vi "MADAQ-SetDACs.vi"(4 "error in (no error)":errorcluster, 5 "DAC 2 [V]":dbl, 6 "DAC  1 [V]":dbl, 7 "VISA resource name":refnum<visa-resource-name>) -> (0 "error out":errorcluster, 3 "VISA resource name out":refnum<visa-resource-name>)   [LabVIEW 2014]
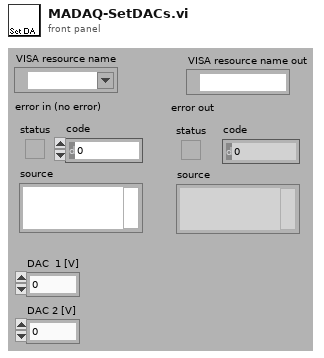
[diagram p1: front panel]
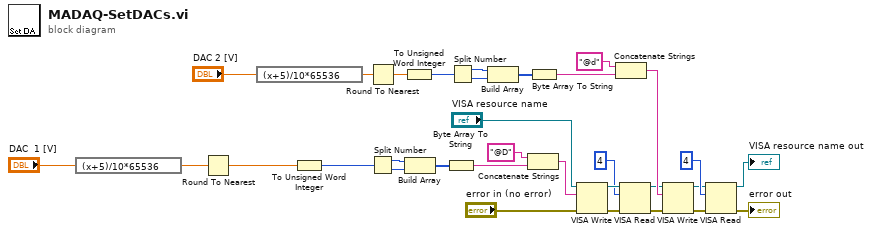
[diagram p0: block diagram]
diagram:
  n1 = expression code="(x+5)/10*65536"("DAC  1 [V]") -> (w8:dbl)
  n2 = Round To Nearest(number=w8) -> (nearest integer value=w7:dbl)
  n3 = expression code="(x+5)/10*65536"("DAC 2 [V]") -> (w6:dbl)
  n4 = To Unsigned Word Integer(number=w7) -> (unsigned 16bit integer=w3:u16)
  n5 = Round To Nearest(number=w6) -> (nearest integer value=w5:dbl)
  n6 = Split Number(x=w3) -> (hi(x)=w32:u8, lo(x)=w31:u8)
  n7 = To Unsigned Word Integer(number=w5) -> (unsigned 16bit integer=w2:u16)
  n8 = Build Array(w32, w31) -> (w28:u8[])
  n9 = Byte Array To String(unsigned byte array=w28) -> (string=w23:string)
  n10 = Split Number(x=w2) -> (hi(x)=w30:u8, lo(x)=w29:u8)
  n11 = Build Array(w30, w29) -> (w27:u8[])
  n12 = Concatenate Strings("@D", w23) -> (w22:string)
  n13 = Byte Array To String(unsigned byte array=w27) -> (string=w11:string)
  n14 = VISA Write(VISA resource name="VISA resource name", write buffer=w22, error in (no error)="error in (no error)") -> (VISA resource name out=w21:refnum<visa-resource-name>, error out=w20:errorcluster)  [unwired: 1 out]
  n15 = Concatenate Strings("@d", w11) -> (w15:string)
  n16 = VISA Read(VISA resource name=w21, byte count=u32 4, error in (no error)=w20) -> (VISA resource name out=w13:refnum<visa-resource-name>, error out=w12:errorcluster)  [unwired: 2 out]
  n17 = VISA Write(VISA resource name=w13, write buffer=w15, error in (no error)=w12) -> (VISA resource name out=w16:refnum<visa-resource-name>, error out=w17:errorcluster)  [unwired: 1 out]
  n18 = VISA Read(VISA resource name=w16, byte count=u32 4, error in (no error)=w17) -> (VISA resource name out=→"VISA resource name out":refnum<visa-resource-name>, error out=→"error out":errorcluster)  [unwired: 2 out]
